vi "Timestamp to ISO8601 Week.vi"(9 "UTC? (F)":bool, 11 "Timestamp (now)":timestamp) -> (1 "ISO8601 Ordinal Date":string, 2 "ISO8601 Weekday":string, 3 "ISO8601 Week":string)   [LabVIEW 2018]
uses:
  <vilib>/Utility/miscctls.llb/LVDateTimeRec.ctl
  isLeapYear (integer).vi
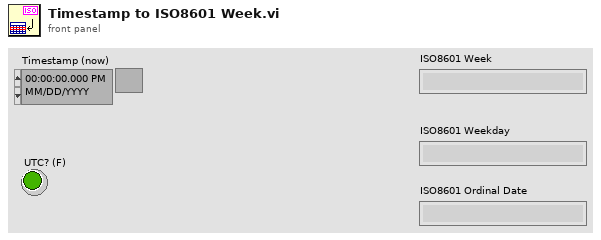
[diagram p1: front panel]
types:
  T1 = typedef "LVDateTimeRec.ctl" = cluster{"fractional second":dbl, "second":i32, "minute":i32, "hour":i32, "day of month":i32, "month":i32, "year":i32, "day of week":i32, "day of year":i32, "DST":i32}
  T2 = typedef "ISO Day -- enum.ctl" = enum16{"Monday", "Tuesday", "Wednesday", "Thursday", "Friday", "Saturday", "Sunday"}
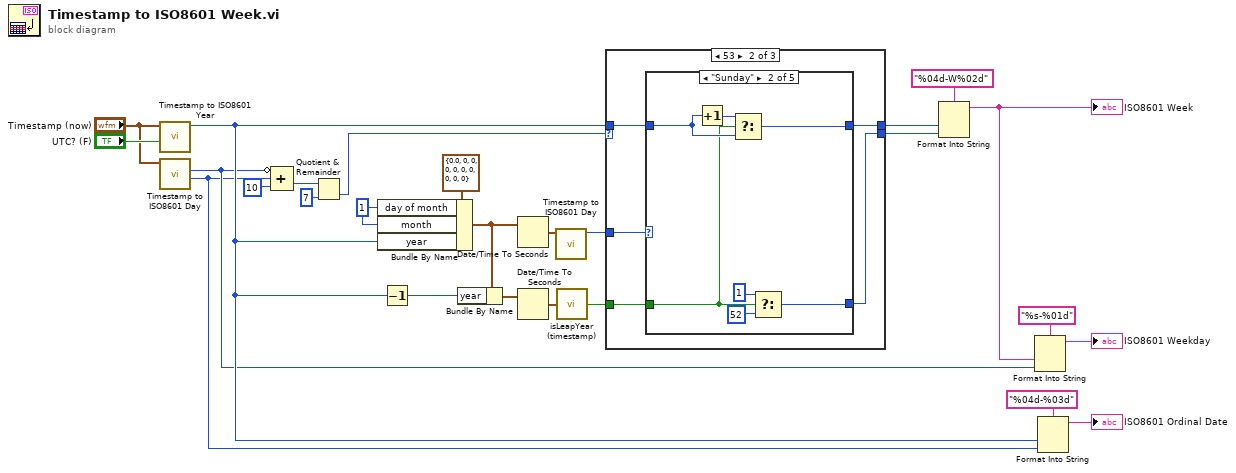
[diagram p0: block diagram]
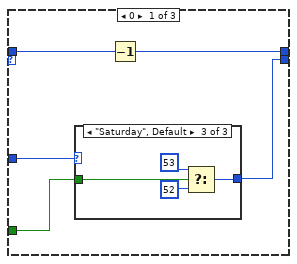
[diagram p2: hidden frame]
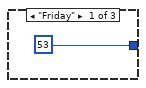
[diagram p3: hidden frame]
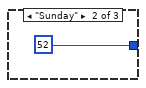
[diagram p4: hidden frame]
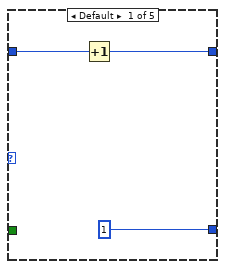
[diagram p5: hidden frame]
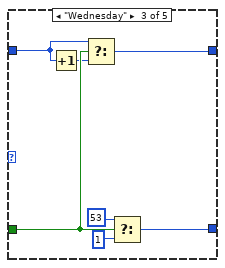
[diagram p6: hidden frame]
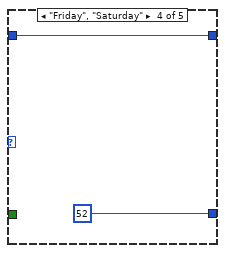
[diagram p7: hidden frame]
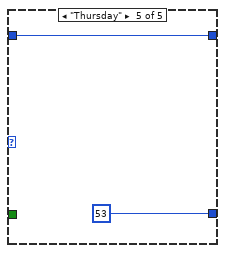
[diagram p8: hidden frame]
diagram:
  w19 = 1 ("day of month")
  n1 = call "Timestamp to ISO8601 Year.vi"("UTC? (F)"="UTC? (F)", "Timestamp (now)"="Timestamp (now)") -> ("year"=w3:i32)  [unwired: 8 in, 1 out]
  n2 = call "Timestamp to ISO8601 Day.vi"("Timestamp (now)"="Timestamp (now)") -> ("Day of Year"=w1:i32, "ISO Weekday"=w2:i32)  [unwired: 8 in, 1 out]
  n3 = Compound Arithmetic op=ADD(invert w2, w1, 10 ("value")) -> (w14:i32)
  n4 = Quotient & Remainder(x=w14, y=7) -> (floor(x/y)=w11:i32)  [unwired: 1 out]
  n5 = Bundle By Name(cluster=T1 {"fractional second"=0.0, "second"=0, "minute"=0, "hour"=0, "day of month"=0, "month"=0, "year"=0, "day of week"=0, "day of year"=0, "DST"=0} ("date time rec"), "day of month"=w19, "month"=w19, "year"=w3) -> (w17:T1)
  n6 = Decrement(x=w3) -> (x-1=w16:i32)
  n7 = Bundle By Name(cluster=w17, "year"=w16) -> (w15:T1)
  n8 = Date/Time To Seconds(2:w17) -> (0:w18:timestamp)  [unwired: 1 in]
  n9 = Date/Time To Seconds(2:w15) -> (0:w10:timestamp)  [unwired: 1 in]
  n10 = call "Timestamp to ISO8601 Day.vi"("Timestamp (now)"=w18) -> ("ISO Day"=w9:T2)  [unwired: 8 in, 2 out]
  n11 = call "isLeapYear (timestamp).vi"("timestamp (now)"=w10) -> ("is Leap Year?"=w8:bool)  [unwired: 8 in]
  n12 = case shown="53" w11 {
    selector: w11 -> [_ _ w64]
    tunnel: [w29 w41 w65] -> w22
    tunnel: w3 -> [w30 w40 w65]
    tunnel: [w31 w42 w64] -> w21
    tunnel: w9 -> [w28 w39 _]
    tunnel: w8 -> [w27 w38 _]
    frame 0 {
      n13 = case shown="\"Saturday\", Default" w28 {
        tunnel: [53 ("year") 52 ("year") w35] -> w31
        tunnel: w27 -> [_ _ w34]
        frame "Friday" {
        }
        frame "Sunday" {
        }
        frame "Saturday", Default {
          n14 = Select(t=53 ("year"), s=w34, f=52 ("year")) -> (s? t:f=w35:i32)
        }
      }
      n15 = Decrement(x=w30) -> (x-1=w29:i32)
    }
    frame 53 {
      n16 = case shown="\"Sunday\"" w39 {
        tunnel: [1 ("year") w50 w57 52 ("year") 53 ("year")] -> w42
        tunnel: [w43 w49 w56 w60 w62] -> w41
        tunnel: w40 -> [w45 w47 w53 w60 w62]
        tunnel: w38 -> [_ w46 w55 _ _]
        frame Default {
          n17 = Increment(x=w45) -> (x+1=w43:i32)
        }
        frame "Sunday" {
          n18 = Increment(x=w47) -> (x+1=w48:i32)
          n19 = Select(t=w48, s=w46, f=w47) -> (s? t:f=w49:i32)
          n20 = Select(t=1 ("year"), s=w46, f=52 ("year")) -> (s? t:f=w50:i32)
        }
        frame "Wednesday" {
          n21 = Increment(x=w53) -> (x+1=w54:i32)
          n22 = Select(t=w53, s=w55, f=w54) -> (s? t:f=w56:i32)
          n23 = Select(t=53 ("year"), s=w55, f=1 ("year")) -> (s? t:f=w57:i32)
        }
        frame "Friday", "Saturday" {
        }
        frame "Thursday" {
        }
      }
    }
    frame Default {
      # "1..52"
    }
  }
  n24 = Format Into String(format string="%04d-W%02d", w22, w21) -> (resulting string=w24:string)  [unwired: 2 in, 1 out]
  "ISO8601 Week" <- w24
  n25 = Format Into String(format string="%s-%01d", w24, w2) -> (resulting string=→"ISO8601 Weekday":string)  [unwired: 2 in, 1 out]
  n26 = Format Into String(format string="%04d-%03d", w3, w1) -> (resulting string=→"ISO8601 Ordinal Date":string)  [unwired: 2 in, 1 out]
